vi "Host_17 - Final.vi"() -> ()   [LabVIEW 2017]
uses:
  <vilib>/Platform/browser.llb/Open URL in Default Browser (string).vi
  <vilib>/Utility/file.llb/Write Delimited Spreadsheet (DBL).vi
panel:
  in  "File Name":path=path "C:/CHIL_SeniorDesign/GUI_Output_Data/CSVdata.csv"
  out "Current (Fixed Scale)":dbl(graph)
  out "Current (Autoscale)":dbl(graph)
  out "Motor Speed (Fixed Scale)":dbl(graph)
  out "Motor Speed (Autoscale)":dbl(graph)
  in  "stop":bool
  out "Current Load Torque":dbl
  out "Current Duty Cycle":dbl
  in  "Duty Cycle (%)":dbl(slide) scale=0.0..100.0
  in  "Load Torque (Nm)":dbl(slide) scale=-0.2..0.2
  in  "Data Update Speed (ms)":dbl
  in  "Website Button":bool
  in  "Doc Button":bool
  in  "Save Button":bool
  # "OPAL-RT Real Time Outputs"
  # "Microcontroller Inputs"
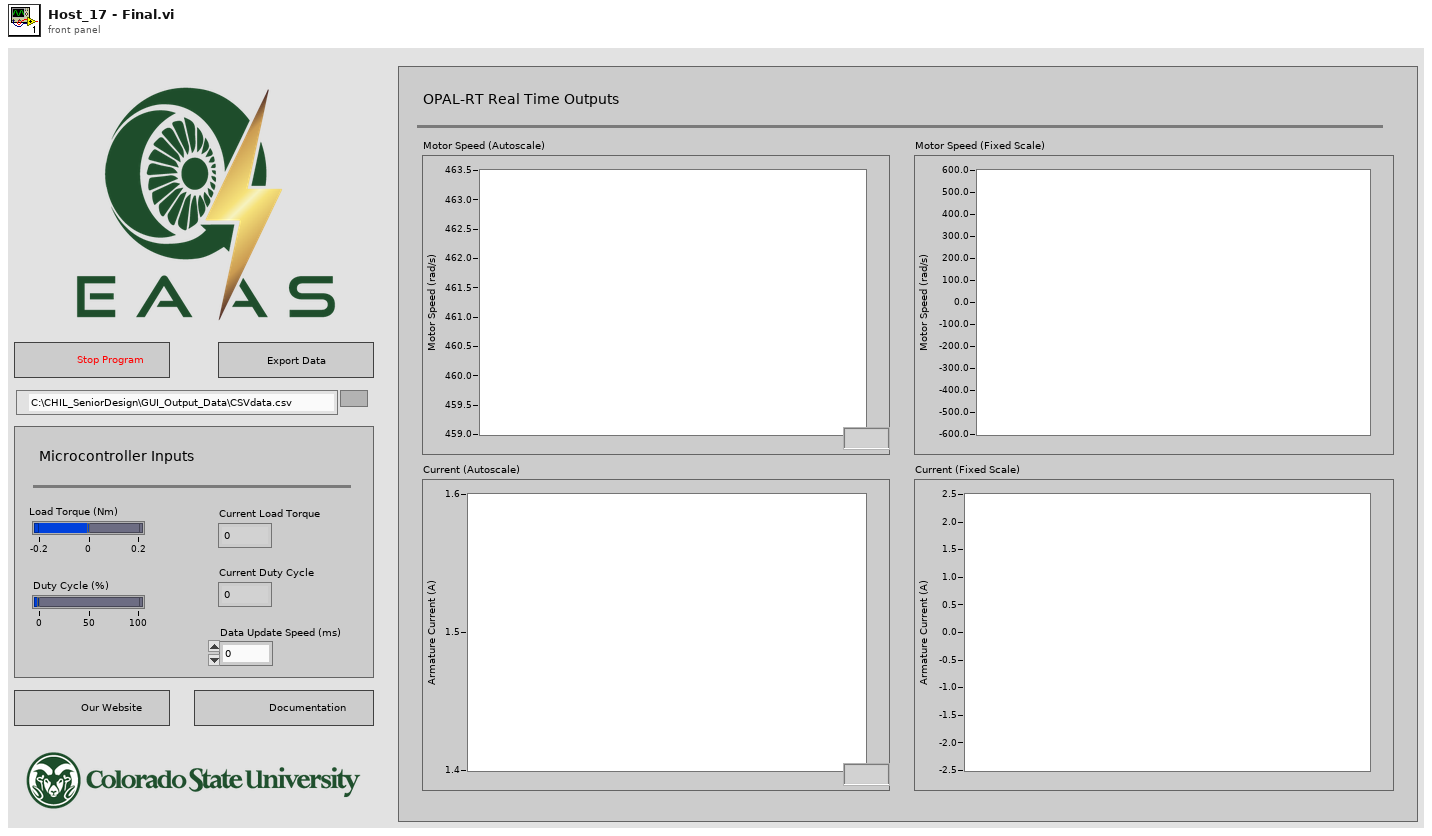
[diagram p1: front panel]
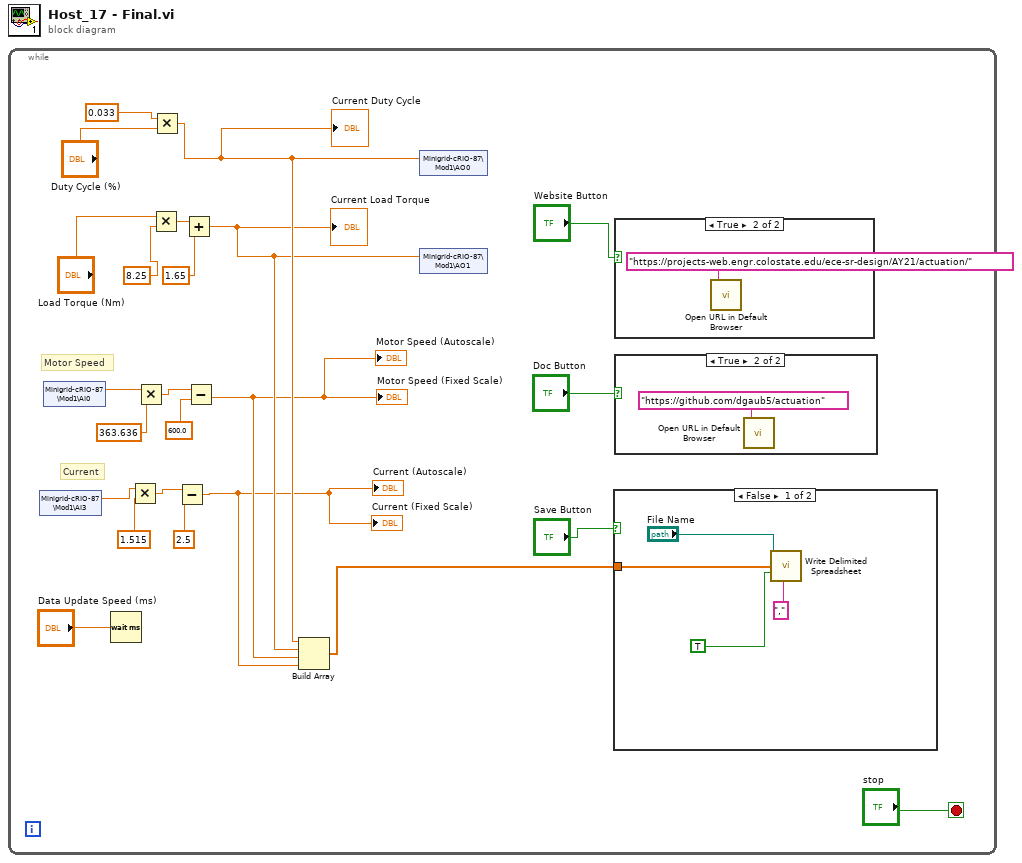
[diagram p0: block diagram]
diagram:
  n1 = while {
    stop <- "stop" stop-if-true
    # "Current"
    # "Motor Speed"
    n2 = shared-variable "Minigrid-cRIO-87\\Mod1\\AI3"() -> (w17:dbl)  [unwired: 1 in, 1 out]
    n3 = shared-variable "Minigrid-cRIO-87\\Mod1\\AI0"() -> (w18:dbl)  [unwired: 1 in, 1 out]
    n4 = Wait (ms)(milliseconds to wait="Data Update Speed (ms)") -> ()  [unwired: 1 out]
    n5 = Multiply(x=w17, y=1.515) -> (x*y=w20:dbl)
    n6 = Multiply(x=w18, y=363.636) -> (x*y=w24:dbl)
    n7 = Multiply(x="Load Torque (Nm)", y=8.25) -> (x*y=w14:dbl)
    n8 = Multiply(x=0.033, y="Duty Cycle (%)") -> (x*y=w4:dbl)
    "Current Duty Cycle" <- w4
    n9 = Subtract(x=w20, y=2.5) -> (x-y=w1:dbl)
    "Current (Autoscale)" <- w1
    "Current (Fixed Scale)" <- w1
    n10 = Add(x=w14, y=1.65) -> (x+y=w3:dbl)
    "Current Load Torque" <- w3
    n11 = Subtract(x=w24, y=600.0) -> (x-y=w2:dbl)
    "Motor Speed (Autoscale)" <- w2
    "Motor Speed (Fixed Scale)" <- w2
    n12 = Build Array(w4, w3, w2, w1) -> (w5:dbl[])
    n13 = shared-variable "Minigrid-cRIO-87\\Mod1\\AO0"(w4) -> ()  [unwired: 1 in, 1 out]
    n14 = shared-variable "Minigrid-cRIO-87\\Mod1\\AO1"(w3) -> ()  [unwired: 1 in, 1 out]
    n15 = case shown="False" "Save Button" {
      tunnel: w5 -> [w26 _]
      frame False {
        n16 = call-poly <vilib>:"Write Delimited Spreadsheet.vi"("file path (dialog if empty)"="File Name", "1D data"=w26, "append to file? (new file:F)"=TRUE, "delimiter (\\t)"="," ("delimiter (\\t)")) -> ()  [unwired: 10 in, 2 out]
      }
      frame True {
      }
    }
    n17 = case shown="True" "Website Button" {
      frame False {
      }
      frame True {
        n18 = call-poly <vilib>:"Open URL in Default Browser.vi"("URL"="https://projects-web.engr.colostate.edu/ece-sr-design/AY21/actuation/") -> ()  [unwired: 5 in, 2 out]
      }
    }
    n19 = case shown="True" "Doc Button" {
      frame False {
      }
      frame True {
        n20 = call-poly <vilib>:"Open URL in Default Browser.vi"("URL"="https://github.com/dgaub5/actuation") -> ()  [unwired: 5 in, 2 out]
      }
    }
  }
